vi "Crosspoint list to pattern.vi"(10 "List":i32[][](array[numeric]), 11 "rows":i32=4) -> (2 "Pattern":u32[](array[numeric]))   [LabVIEW 2020, in "Pickering.lvlib" / "PIPX40 Matrix.lvclass"]
uses:
  PIPX40 Matrix.lvclass
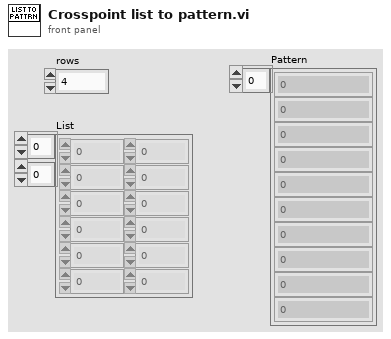
[diagram p1: front panel]
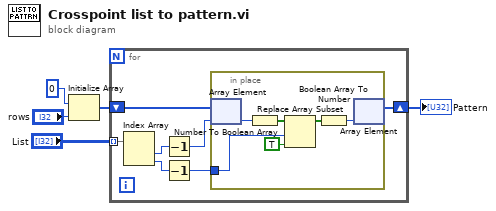
[diagram p0: block diagram]
diagram:
  n1 = Initialize Array(u32 0, "rows") -> (w2:u32[])
  n2 = for {
    tunnel: "List" -> [w12] mode=indexing
    shift-right: [w8] -> w1
    shift-left: w2 -> [w11]
    n3 = Index Array(array=w12) -> (element #1=w9:i32, element #2=w10:i32)  [unwired: 2 in]
    n4 = Decrement(x=w9) -> (x-1=w7:i32)
    n5 = Decrement(x=w10) -> (x-1=w6:i32)
    n6 = in-place {
      in-place-border: w6 -> [w15]
      n7 = in-place-array #1(w11, w7) -> (w18:u32)
      n8 = Number To Boolean Array(number=w18) -> (Boolean array=w14:bool[])
      n9 = Replace Array Subset(array=w14, new element=TRUE, index=w15) -> (w13:bool[])
      n10 = Boolean Array To Number(Boolean array=w13) -> (number=w16:u32)
      n11 = in-place-array #1(w16) -> (w8:u32[])  [unwired: 1 out]
    }
  }
  "Pattern" <- w1
